vi "Read State PMG.vi"(0 "Pump_1AI_1DO_2DI in":refnum<class "PM_Group.lvclass">) -> (6 "State PMG":T2, 8 "State M12":T1, 10 "State M21":T1, 15 "State M24":T1)   [LabVIEW 2019, in "PM_Group.lvclass"]
uses:
  PM_Group.lvclass
  TypeDef/State PMG.ctl
  TypeDef/State Engine.ctl
  PM_Group.lvclass/PM_Group.ctl
  Engine_1DO_2DI_class/Engine_1DO_2DI.lvclass/Engine_1DO_2DI.ctl
  Engine_1DO_2DI_class/Engine_1DO_2DI.lvclass
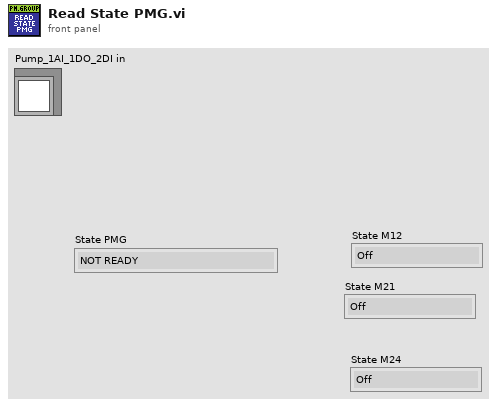
[diagram p1: front panel]
types:
  T1 = typedef "State Engine.ctl" = enum16{"Off", "TupningOn", "On", "TurningOff"}
  T2 = typedef "State PMG.ctl" = enum16{"NOT READY", "IDLE", "ACTIVE", "ERROR"}
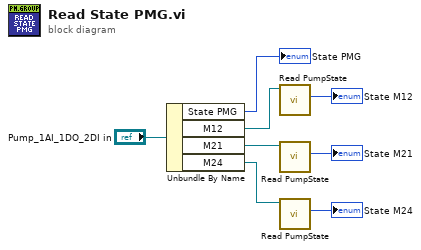
[diagram p0: block diagram]
diagram:
  n1 = Unbundle By Name("Pump_1AI_1DO_2DI in") -> ("State PMG"=→"State PMG":T2, "M12"=w6:refnum<class "Engine_1DO_2DI.lvclass">, "M21"=w2:refnum<class "Engine_1DO_2DI.lvclass">, "M24"=w1:refnum<class "Engine_1DO_2DI.lvclass">)
  n2 = call "Read PumpState.vi"("Pump_1AI_1DO_2DI in"=w6) -> ("PumpState"=→"State M12":T1)  [unwired: 10 in]
  n3 = call "Read PumpState.vi"("Pump_1AI_1DO_2DI in"=w2) -> ("PumpState"=→"State M21":T1)  [unwired: 10 in]
  n4 = call "Read PumpState.vi"("Pump_1AI_1DO_2DI in"=w1) -> ("PumpState"=→"State M24":T1)  [unwired: 10 in]
